vi "Check_Input.vi"(8 "error in":errorcluster, 11 "Diameter (in)":dbl[](array[numeric])) -> (0 "error out":errorcluster)   [LabVIEW 2025]
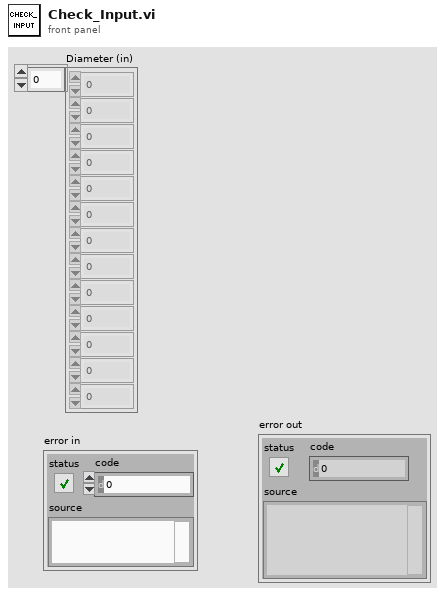
[diagram p1: front panel]
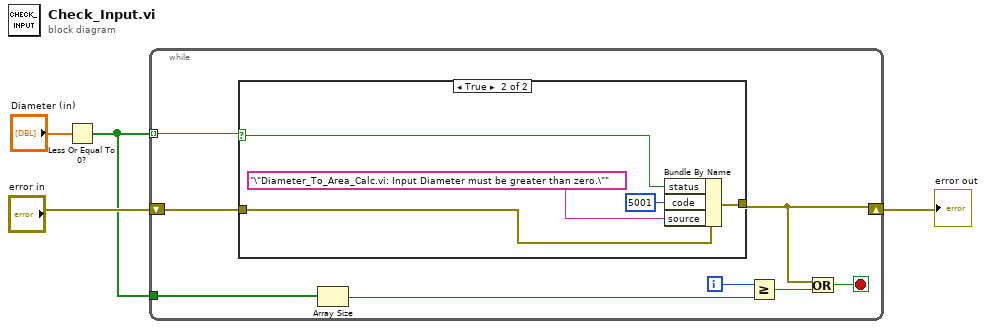
[diagram p0: block diagram]
diagram:
  n1 = Less Or Equal To 0?(x="Diameter (in)") -> (x <= 0?=w1:bool[])
  n2 = while {
    shift-right: [w8] -> w2
    shift-left: "error in" -> [w12]
    tunnel: w1 -> [w11] mode=indexing
    tunnel: w1 -> [w10]
    i -> [w7]
    stop <- w9 stop-if-true
    n3 = case shown="True" w11 {
      selector: w11 -> [_ w16]
      tunnel: w12 -> [w13 w18]
      tunnel: [w13 w17] -> w8
      frame False {
      }
      frame True {
        n4 = Bundle By Name(cluster=w18, "status"=w16, "code"=5001, "source"="\"Diameter_To_Area_Calc.vi: Input Diameter must be greater than zero.\"") -> (w17:errorcluster)
      }
    }
    n5 = Array Size(array=w10) -> (size(s)=w5:i32)
    n6 = Greater Or Equal?(x=w7, y=w5) -> (x >= y?=w6:bool)
    n7 = Or(x=w8, y=w6) -> (x .or. y?=w9:bool)
  }
  "error out" <- w2
